vi "Read dotNET Custom Action Definitions.vi"(8 "error in (no error)":errorcluster, 10 "Custom Action Definitions":refnum<k24>[](array[refnum]), 11 "Bundle Builder in":refnum<class "Bundle Builder.lvclass">) -> (0 "error out":errorcluster, 3 "Bundle Builder out":refnum<class "Bundle Builder.lvclass">)   [LabVIEW 2020, in "Bundle Builder.lvclass"]
uses:
  Bundle Builder.lvclass
  Bundle Builder.lvclass/Bundle Builder.ctl
  C:/Users/chihong/Documents/Repos/StsCustomBundleBuilder/Code/StsCustomBundleBuilderLib/StsCustomBundleBuilderLib/bin/Debug/StsCustomBundleBuilderLib.dll
  StsCustomBundleBuilderLib/StsCustomBundleBuilderLib/bin/Debug/StsCustomBundleBuilderLib.dll
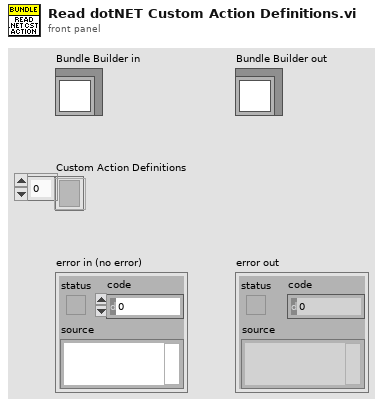
[diagram p1: front panel]
types:
  T1 = cluster{"Display Name":string, "Commands":cluster{"Path":string, "Parameters":string, "Successful Exit Codes":string, "Log Command":cluster{"Flag":string, "File Name":string}}[]}
  T2 = cluster{"Path":string, "Parameters":string, "Successful Exit Codes":string, "Log Command":cluster{"Flag":string, "File Name":string}}
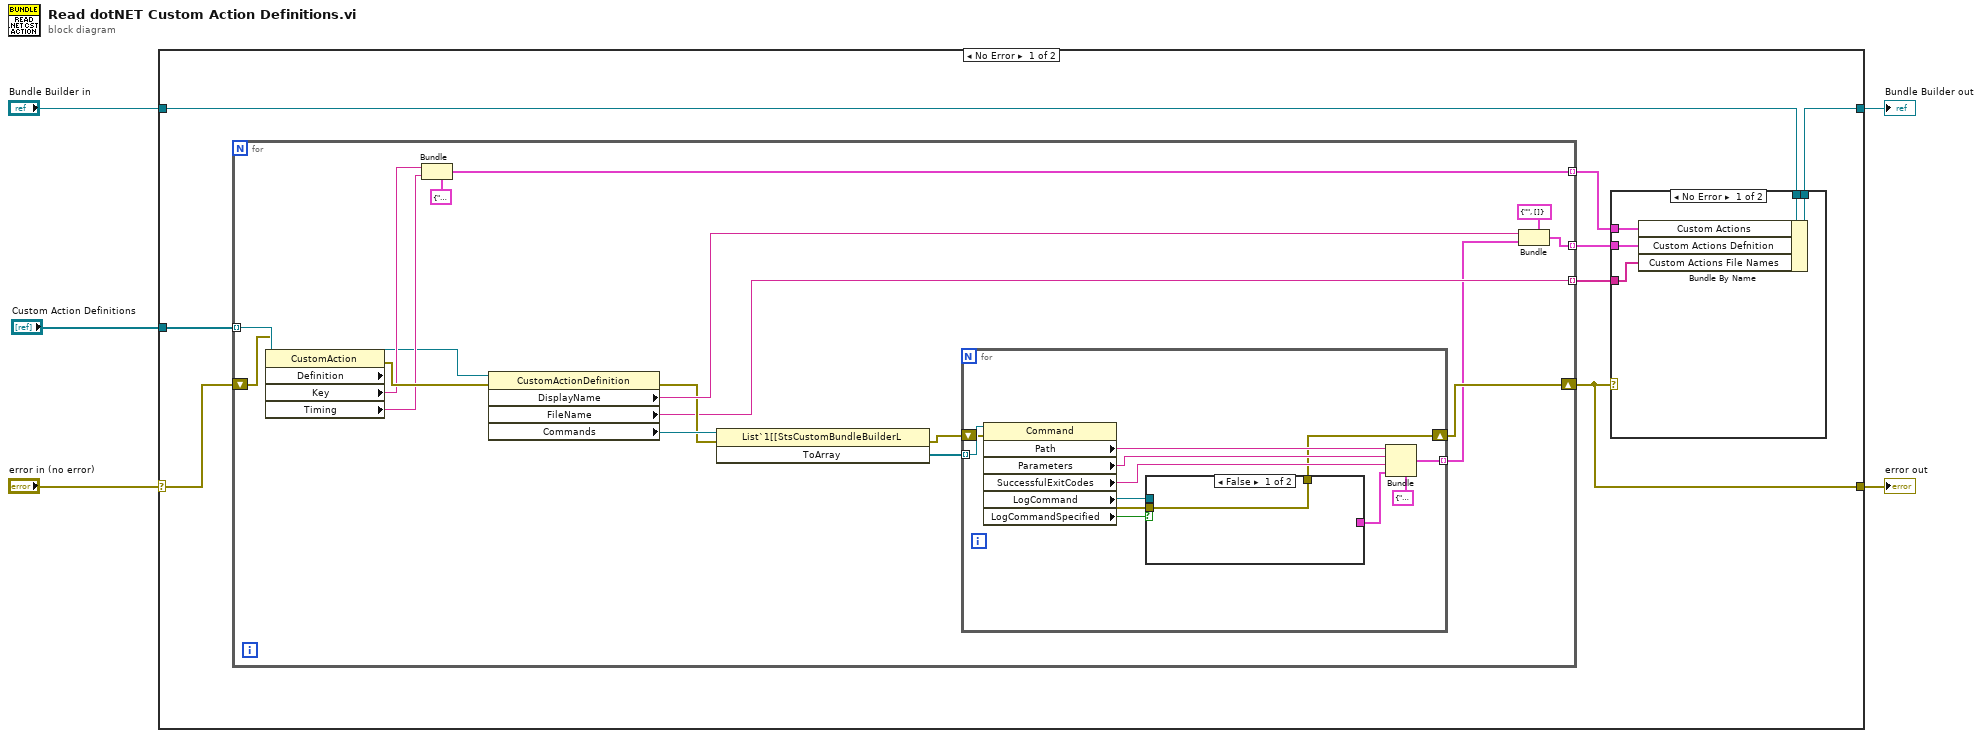
[diagram p0: block diagram]
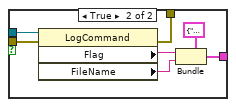
[diagram p3: hidden frame]
diagram:
  n1 = case shown="No Error" "error in (no error)" {
    selector: "error in (no error)" -> [w11 w59]
    tunnel: [w7 w59] -> w4
    tunnel: [w10 w58] -> w2
    tunnel: "Bundle Builder in" -> [w13 w58]
    tunnel: "Custom Action Definitions" -> [w12 _]
    frame No Error {
      n2 = for {
        tunnel: w12 -> [w37] mode=indexing
        shift-right: [w26] -> w7
        shift-left: w11 -> [w36]
        tunnel: [w25] -> w9 mode=indexing
        tunnel: [w24] -> w8 mode=indexing
        tunnel: [w23] -> w6 mode=indexing
        n3 = property class="CustomAction"(reference=w37, error in=w36) -> (error out=w35:errorcluster, "Definition"=w32:refnum<k24>, "Key"=w34:string, "Timing"=w33:string)  [unwired: 1 out]
        n4 = Bundle(cluster=cluster{"Key":string, "Timing":string} {"Key"="", "Timing"=""} ("Product Installer"), "Key"=w34, "Timing"=w33) -> (w24:cluster{"Key":string, "Timing":string})
        n5 = property class="CustomActionDefinition"(reference=w32, error in=w35) -> (error out=w29:errorcluster, "DisplayName"=w31:string, "FileName"=w23:string, "Commands"=w30:refnum<k24>)  [unwired: 1 out]
        n6 = invoke class="List`1[[StsCustomBundleBuilderL" method="ToArray"(reference=w30, error in=w29) -> (error out=w27:errorcluster, "ToArray"=w28:refnum<k24>[])  [unwired: 1 in, 1 out]
        n7 = for {
          tunnel: w28 -> [w49] mode=indexing
          tunnel: [w41] -> w20 mode=indexing
          shift-right: [w40] -> w26
          shift-left: w27 -> [w44]
          n8 = property class="Command"(reference=w49, error in=w44) -> (error out=w45:errorcluster, "Path"=w47:string, "Parameters"=w46:string, "SuccessfulExitCodes"=w43:string, "LogCommand"=w39:refnum<k24>, "LogCommandSpecified"=w38:bool)  [unwired: 1 out]
          n9 = case shown="False" w38 {
            tunnel: w45 -> [w50 w57]
            tunnel: [_ w55] -> w42
            tunnel: [w50 w52] -> w40
            tunnel: w39 -> [_ w51]
            frame False {
            }
            frame True {
              n10 = property class="LogCommand"(reference=w51, error in=w57) -> (error out=w52:errorcluster, "Flag"=w54:string, "FileName"=w53:string)  [unwired: 1 out]
              n11 = Bundle(cluster=cluster{"Flag":string, "File Name":string} {"Flag"="", "File Name"=""} ("Log Command"), "Flag"=w54, "File Name"=w53) -> (w55:cluster{"Flag":string, "File Name":string})
            }
          }
          n12 = Bundle(cluster=T2 {"Path"="", "Parameters"="", "Successful Exit Codes"="", "Log Command"={"Flag"="", "File Name"=""}} ("Product Installer"), "Path"=w47, "Parameters"=w46, "Successful Exit Codes"=w43, "Log Command"=w42) -> (w41:T2)
        }
        n13 = Bundle(cluster=T1 {"Display Name"="", "Commands"=[]} ("Custom Actions"), "Display Name"=w31, "Commands"=w20) -> (w25:T1)
      }
      n14 = case shown="No Error" w7 {
        tunnel: w13 -> [w18 w19]
        tunnel: [w17 w19] -> w10
        tunnel: w9 -> [w14 _]
        tunnel: w8 -> [w16 _]
        tunnel: w6 -> [w15 _]
        frame No Error {
          n15 = Bundle By Name(cluster=w18, "Custom Actions"=w16, "Custom Actions Defnition"=w14, "Custom Actions File Names"=w15) -> (w17:refnum<class "Bundle Builder.lvclass">)
        }
        frame Error {
        }
      }
    }
    frame Error {
    }
  }
  "error out" <- w4
  "Bundle Builder out" <- w2
